vi "U16ToU8ArrayBigendian(SubVI).vi"(11 "int data":u16 format="%x") -> (2 "low byte":u8 format="%x", 3 "high byte":u8 format="%x")   [LabVIEW 2012]
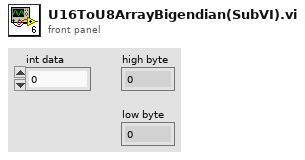
[diagram p1: front panel]
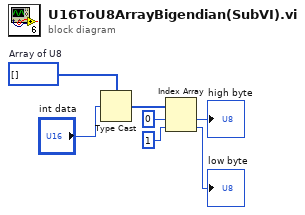
[diagram p0: block diagram]
diagram:
  w1 = u8[] []  # Array of U8
  n1 = Type Cast(type=w1, x="int data") -> (*(type *) &x=w2:u8[])
  n2 = Index Array(array=w2, index #1=0, index #2=1) -> (element #1=→"high byte":u8, element #2=→"low byte":u8)
